vi "Stop Test using Abs.vi"(8 "error in (no error)":errorcluster, 10 "Stop Test":bool, 11 "User Interface in":refnum<class "User Interface.lvclass">) -> (0 "error out":errorcluster, 3 "User Interface out":refnum<class "User Interface.lvclass">)   [LabVIEW 2017, in "User Interface.lvlib" / "User Interface.lvclass"]
uses:
  User Interface.lvclass
  C:/Program Files (x86)/National Instruments/LabVIEW 2017/vi.lib/ActorFramework/Actor/Actor.lvclass
  <vilib>/ActorFramework/Actor/Actor.lvclass/Actor.ctl
  User Interface.lvclass/User Interface.ctl
  User Interface Messages/Stop Test Msg/Stop Test Msg.lvclass/Stop Test Msg.ctl
  <vilib>/ActorFramework/Message Enqueuer/Message Enqueuer.lvclass/Message Enqueuer.ctl
  <vilib>/ActorFramework/Message Enqueuer/Enqueue.vi
  User Interface Messages/Stop Test Msg/Stop Test Msg.lvclass
  C:/Program Files (x86)/National Instruments/LabVIEW 2017/vi.lib/ActorFramework/Message/Message.lvclass
  <vilib>/ActorFramework/Message Priority Queue/Priority Enqueue.vi
  <vilib>/ActorFramework/Actor/Actor.lvclass
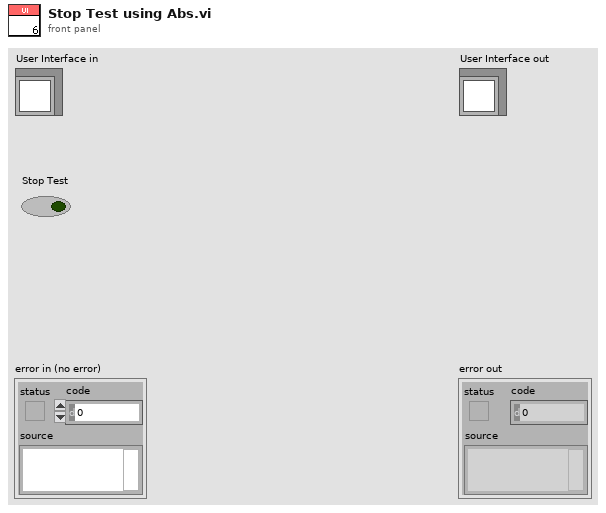
[diagram p1: front panel]
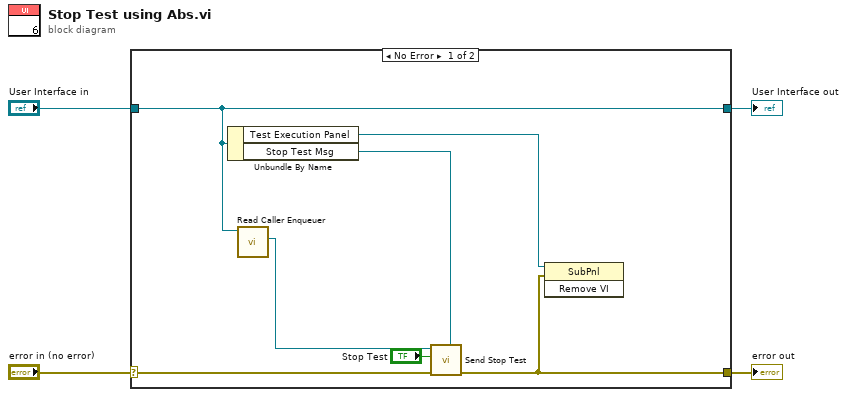
[diagram p0: block diagram]
diagram:
  n1 = case shown="No Error" "error in (no error)" {
    selector: "error in (no error)" -> [w11 w13]
    tunnel: [w5 w13] -> w3
    tunnel: [w10 w12] -> w1
    tunnel: "User Interface in" -> [w10 w12]
    frame No Error {
      n2 = Unbundle By Name(w10) -> ("Test Execution Panel"=w6:refnum<vi>, "Stop Test Msg"=w8:refnum<class "Stop Test Msg.lvclass">)
      n3 = call <vilib>:"Read Caller Enqueuer.vi"("Actor"=w10) -> ("Caller Enqueuer"=w9:refnum<class "Message Enqueuer.lvclass">)  [unwired: 10 in]
      n4 = call "Send Stop Test.vi"("Message Type"=w8, "error in (no error)"=w11, "Stop Test"="Stop Test", "Message Enqueuer"=w9) -> ("error out"=w5:errorcluster)  [unwired: 6 in, 1 out]
      n5 = invoke class="SubPnl" method="Remove VI"(reference=w6, error in=w5) -> ()  [unwired: 1 in, 3 out]
    }
    frame Error {
    }
  }
  "error out" <- w3
  "User Interface out" <- w1
